vi "Read Industrial Port Edge Detection.vi"() -> ()   [LabVIEW 8.6]
uses:
  vi.lib/UeiDaq/UeiDaqReadOneDigitalScanUInt16.vi
  vi.lib/UeiDaq/UeiDaqReadOneDigitalScanUInt32.vi
  vi.lib/UeiDaq/UeiDaqCreateDIIndustrialSession.vi
  <libdir>/resource/objmgr/ueidaq.rc
panel:
  out "Timeout occurred":bool
  in  "Timeout (ms)":u32
  in  "Edge Masks":u32[](array[numeric])
  in  "Digital filter min.\n input width (ms)":dbl
  in  "High Threshold":dbl
  in  "Low Threshold":dbl
  out "device name":string
  out "DI Resolution (bits)":u32
  out "Raw Data":i32[](array[numeric]) format="%x"
  out "DI ports":bool[][](array[boolean])
  in  "DI Resource":string
  out "Total scans acquired":u32
  in  "stop":bool
  # "READ FROM DIGITAL IN (Point by Point)"
  # "1/ Set the resource name -->"
  # "2/ Set the input port parameters -->"
  # "Device info"
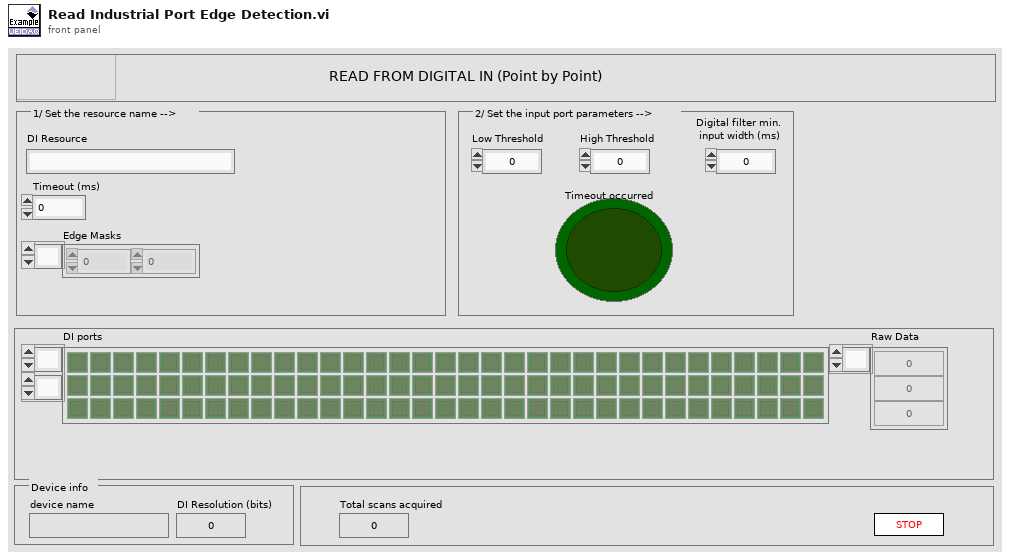
[diagram p1: front panel]
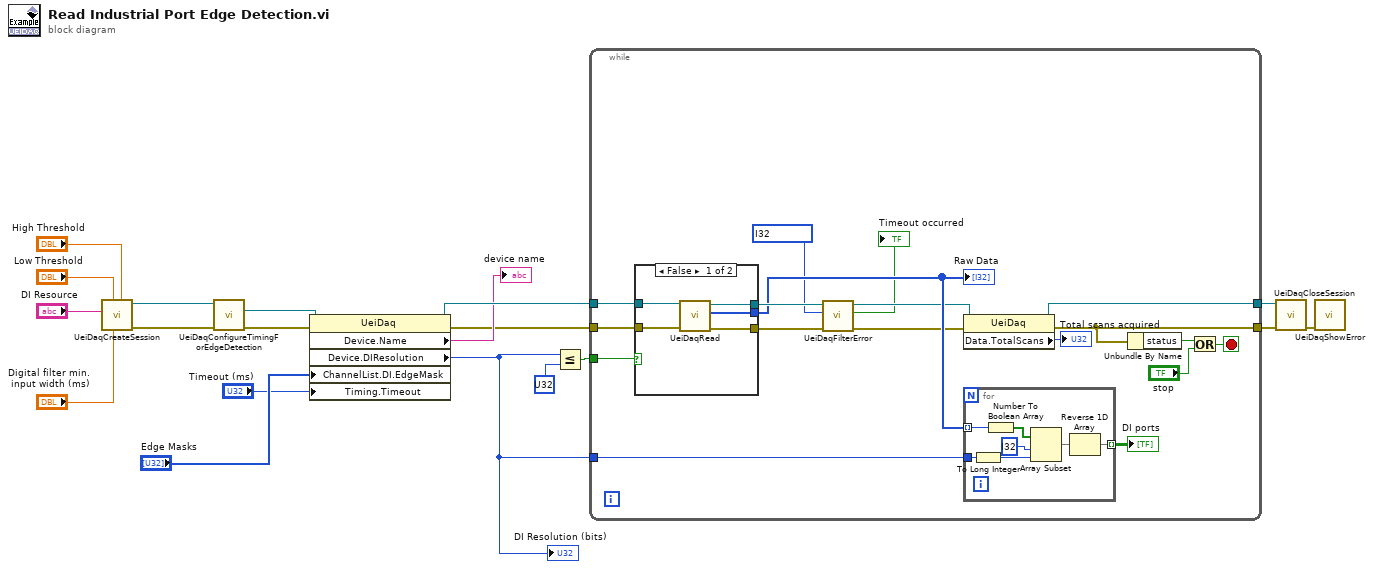
[diagram p0: block diagram]
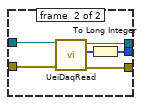
[diagram p2: hidden frame]
diagram:
  n1 = call-poly "UeiDaqCreateSession.vi"("High Threshold"="High Threshold", "Minimum pulse width"="Digital filter min.\n input width (ms)", "Low Threshold"="Low Threshold", "Resource"="DI Resource") -> ("error out"=w17:errorcluster, "UeiDaq Refnum Out"=w18:refnum<k20>)  [unwired: 2 in, 4 out]
  n2 = call "UeiDaqConfigureTimingForEdgeDetection.vi"("error in (no error)"=w17, "UeiDaq Refnum In"=w18) -> ("error out"=w13:errorcluster, "UeiDaq Refnum Out"=w15:refnum<k20>)  [unwired: 8 in]
  n3 = property class="UeiDaq"(reference=w15, error in=w13, "ChannelList.DI.EdgeMask"="Edge Masks", "Timing.Timeout"="Timeout (ms)") -> (reference out=w14:refnum<k20>, error out=w3:errorcluster, "Device.Name"=→"device name":string, "Device.DIResolution"=w8:u32)
  "DI Resolution (bits)" <- w8
  n4 = Less Or Equal?(x=w8, y=u32 ?) -> (x <= y?=w11:bool)
  n5 = while {
    tunnel: w14 -> [w29]
    tunnel: w11 -> [w27]
    tunnel: [w37] -> w9
    tunnel: w8 -> [w31]
    tunnel: w3 -> [w28]
    tunnel: [w33] -> w10
    stop <- w32 stop-if-true
    n6 = case shown="False" w27 {
      tunnel: [w42 w47] -> w23
      tunnel: [w41 w46] -> w26
      tunnel: [w40 w45] -> w25
      tunnel: w29 -> [w39 w44]
      tunnel: w28 -> [w38 w43]
      frame #0 {
        n7 = call-poly "UeiDaqRead.vi"("error in (no error)"=w38, "UeiDaq Refnum In"=w39) -> ("error out"=w42:errorcluster, "Raw Data"=w40:i32[], "UeiDaq Refnum Out"=w41:refnum<k20>)  [unwired: 7 out]
      }
      frame #1 {
        n8 = call-poly "UeiDaqRead.vi"("error in (no error)"=w43, "UeiDaq Refnum In"=w44) -> ("error out"=w47:errorcluster, "Raw Data"=w48:i16[], "UeiDaq Refnum Out"=w46:refnum<k20>)  [unwired: 7 out]
        n9 = To Long Integer(number=w48) -> (32bit integer=w45:i32[])
      }
    }
    "Raw Data" <- w25
    n10 = call "UeiDaqFilterError.vi"("error in (no error)"=w23, "Error to filter"=i32 ?, "UeiDaq Refnum In"=w26) -> ("error out"=w22:errorcluster, "Error filtered"=→"Timeout occurred":bool, "UeiDaq Refnum Out"=w24:refnum<k20>)  [unwired: 6 in]
    n11 = property class="UeiDaq"(reference=w24, error in=w22) -> (reference out=w37:refnum<k20>, error out=w33:errorcluster, "Data.TotalScans"=→"Total scans acquired":u32)
    n12 = for {
      tunnel: w31 -> [w53]
      tunnel: [w51] -> w30 mode=indexing
      tunnel: w25 -> [w49] mode=indexing
      n13 = To Long Integer(number=w53) -> (32bit integer=w50:i32)
      n14 = Number To Boolean Array(number=w49) -> (Boolean array=w55:bool[])
      n15 = Array Subset(array=w55, index=i32 ?, length=w50) -> (w52:bool[])
      n16 = Reverse 1D Array(array=w52) -> (reversed array=w51:bool[])
    }
    "DI ports" <- w30
    n17 = Unbundle By Name(w33) -> ("status"=w35:bool)
    n18 = Or(x=w35, y="stop") -> (x .or. y?=w32:bool)
  }
  n19 = call "UeiDaqCloseSession.vi"("error in (no error)"=w10, "UeiDaq Refnum In"=w9) -> ("error out"=w19:errorcluster)  [unwired: 1 in, 8 out]
  n20 = call "UeiDaqShowError.vi"("error in (no error)"=w19) -> ()  [unwired: 2 in, 9 out]
